vi "DelimiterToStringRepresentation.vi"(10 "Delimiter":refnum<class "Delimiter.lvclass">) -> (2 "String representation":string)   [LabVIEW 2014, in "Delimiter.lvclass"]
uses:
  Delimiter.lvclass
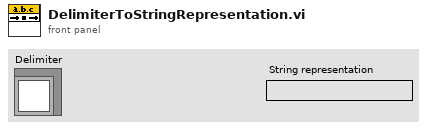
[diagram p1: front panel]
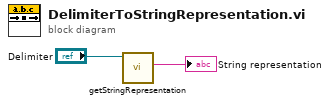
[diagram p0: block diagram]
diagram:
  n1 = call-dynamic "getStringRepresentation.vi"("Delimiter in"="Delimiter") -> ("String representation"=→"String representation":string)  [unwired: 9 in, 1 out]
